vi "niDDC Set DDC parameters.vi"(7 "input.gain":T1={"gain I"=0.0, "gain Q"=1.0} {"gain I" format="%.22g"; "gain Q" format="%.22g"}, 8 "error in (no error)":errorcluster, 9 "DDC IQ rates (Hz)":dbl[](array[numeric])=[1000000.0] format="%#_6p", 10 "DDC Freq shift (Hz)":dbl[](array[numeric])=[50.0] format="%_5p", 11 "Class in":refnum<class "7976R_v1.lvclass">) -> (0 "error out":errorcluster, 3 "Class out":refnum<class "7976R_v1.lvclass">)   [LabVIEW 2015, in "7976R_v1.lvclass"]
uses:
  <userlib>/SE-APP-Receiver/NI5772/7976R_v1/7976R_v1.lvclass
  <userlib>/SE-APP-Receiver/NI5772/7976R_v1/7976R_v1.lvclass/7976R_v1.ctl
  <vilib>/Utility/error.llb/Error Cluster From Error Code.vi
  <vilib>/rvi/errors/niLvFpgaAdjustHostInterfaceError.vi
  <vilib>/rvi/interface/nirviReadWriteControl/nirviReadWriteControl.xnode
  <userlib>/SE-APP-Receiver/NI5772/7976R_v1/Private/FPGA VI Reference_DDC_v1.8.ctl
  NiFpgaLv.dll
  <vilib>/rvi/interface/Simulation/niFpgaSimulationCallBeginRW.vi
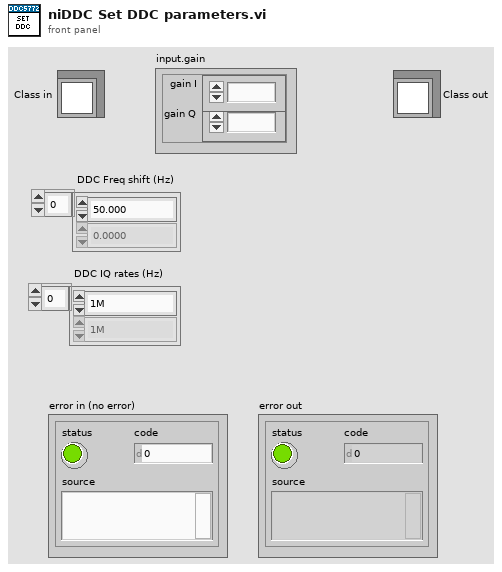
[diagram p1: front panel]
types:
  T1 = cluster{"gain I":fxp<+/-,24,3>, "gain Q":fxp<+/-,24,3>}
  T2 = typedef "7976R_v1.lvclass/FPGA VI Reference_DDC_v1.8.ctl" = refnum<k20>
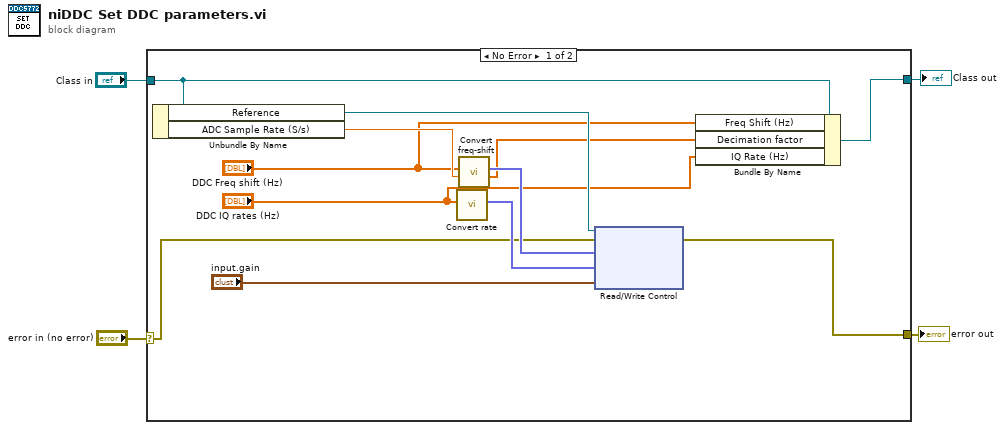
[diagram p0: block diagram]
diagram:
  n1 = case shown="No Error" "error in (no error)" {
    selector: "error in (no error)" -> [w14 w18]
    tunnel: [w13 w18] -> w4
    tunnel: "Class in" -> [w8 w17]
    tunnel: [w7 w17] -> w1
    frame No Error {
      n2 = Unbundle By Name(w8) -> ("Reference"=w12:T2, "ADC Sample Rate (S/s)"=w10:dbl)
      n3 = call <userlib>:"Convert rate.vi"("DDC IQ rates (kHz)"="DDC IQ rates (Hz)") -> ("ddc.out.rate"=w16:fxp<+,48,1>[])  [unwired: 10 in]
      n4 = call <userlib>:"Convert freq-shift.vi"("ADC Sample Rate [Hz]"=w10, "Frequency Shift (Hz)"="DDC Freq shift (Hz)") -> ("Decimation Factor"=w9:dbl[], "ddc.freq.shift"=w15:fxp<+/-,48,0>[])  [unwired: 8 in]
      n5 = xnode "Read/Write Control"("FPGA VI Reference In"=w12, "error in"=w14, "ddc.freq.shift"=w15, "ddc.out.rate"=w16, "input.gain"="input.gain") -> ("error out"=w13:errorcluster)  [unwired: 1 out]
      n6 = Bundle By Name(cluster=w8, "Freq Shift (Hz)"="DDC Freq shift (Hz)", "Decimation factor"=w9, "IQ Rate (Hz)"="DDC IQ rates (Hz)") -> (w7:refnum<class "7976R_v1.lvclass">)
    }
    frame Error {
    }
  }
  "error out" <- w4
  "Class out" <- w1
